vi "GetOutputEnableState.vi"(8 "Error In":errorcluster, 11 "Keithley 6482 In":refnum<visa-resource-name>) -> (0 "Error Out":errorcluster, 2 "Enabled?":bool, 3 "Keithley 6482 Out":refnum<visa-resource-name>)   [LabVIEW 2009, in "Keithley-6482-Visa.lvlib"]
uses:
  <instrlib>/Keithley-6482-Visa9.0/Keithley-6482-Visa.lvlib
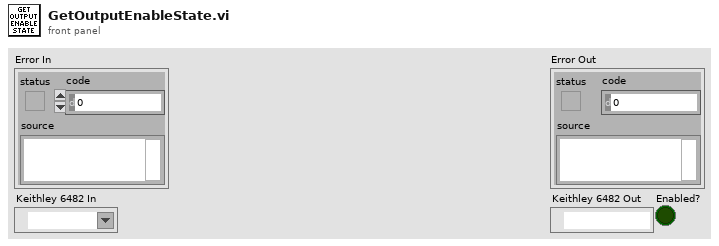
[diagram p1: front panel]
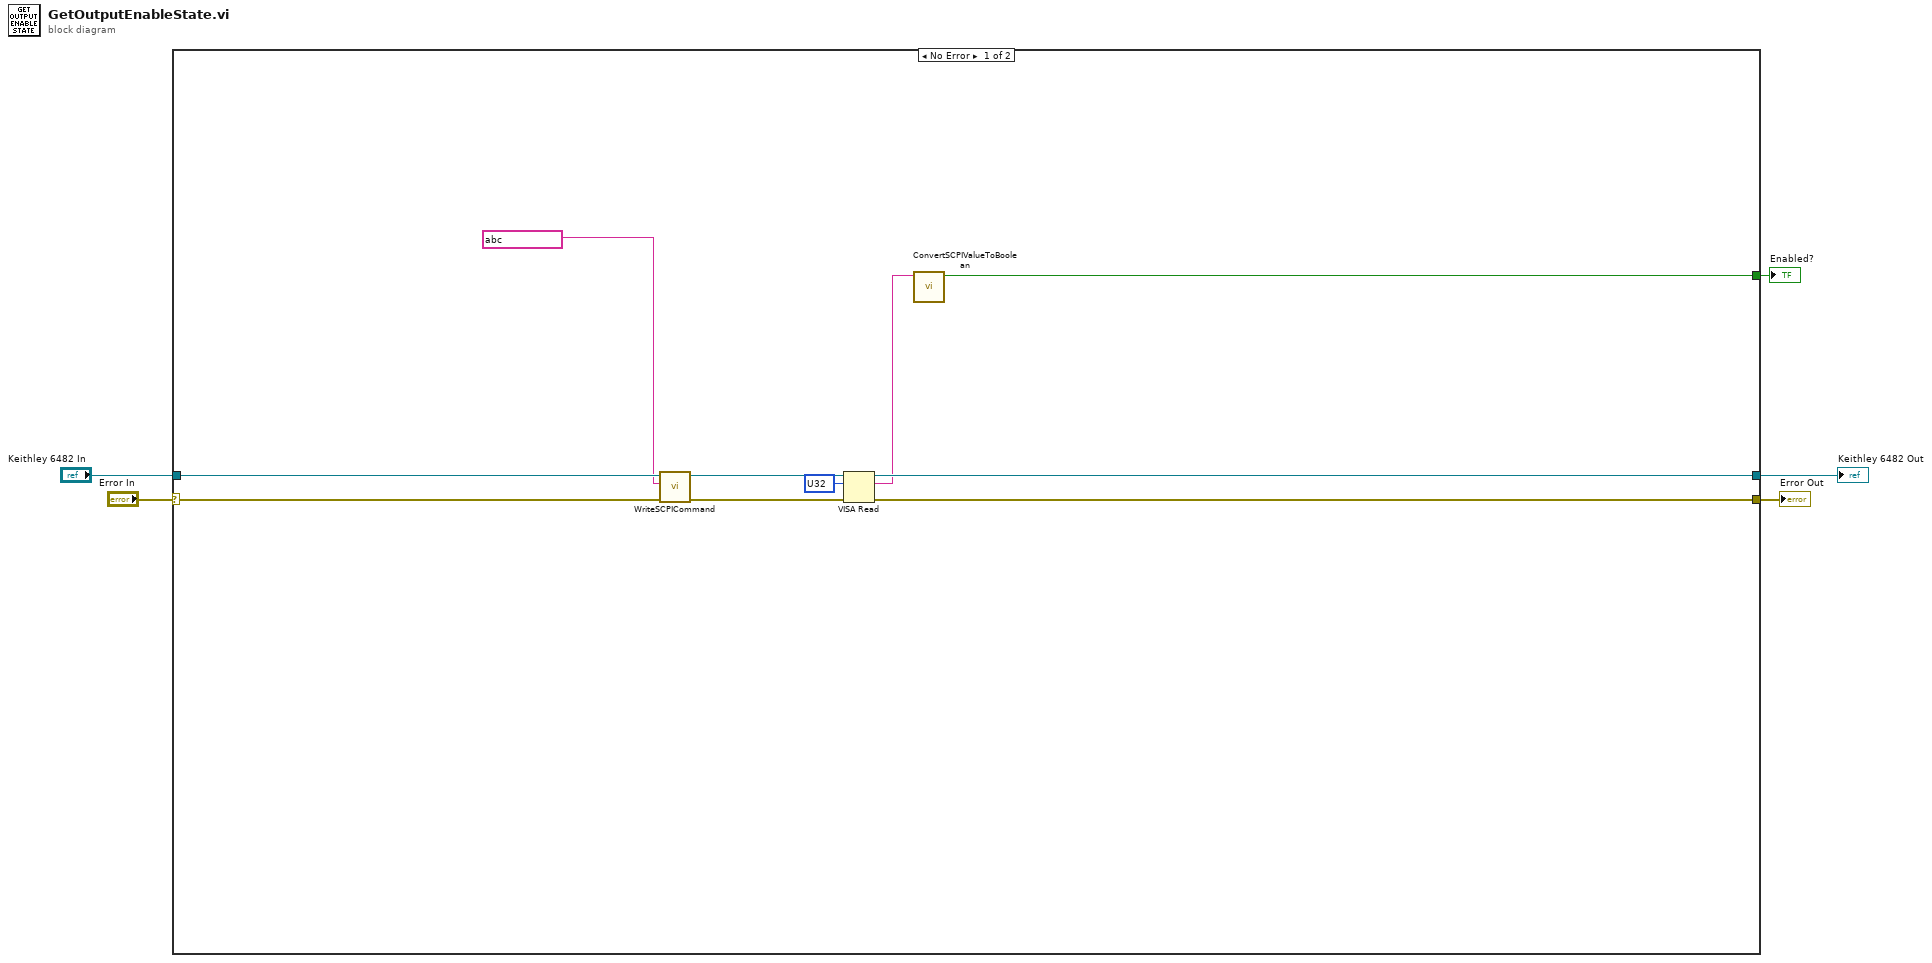
[diagram p0: block diagram]
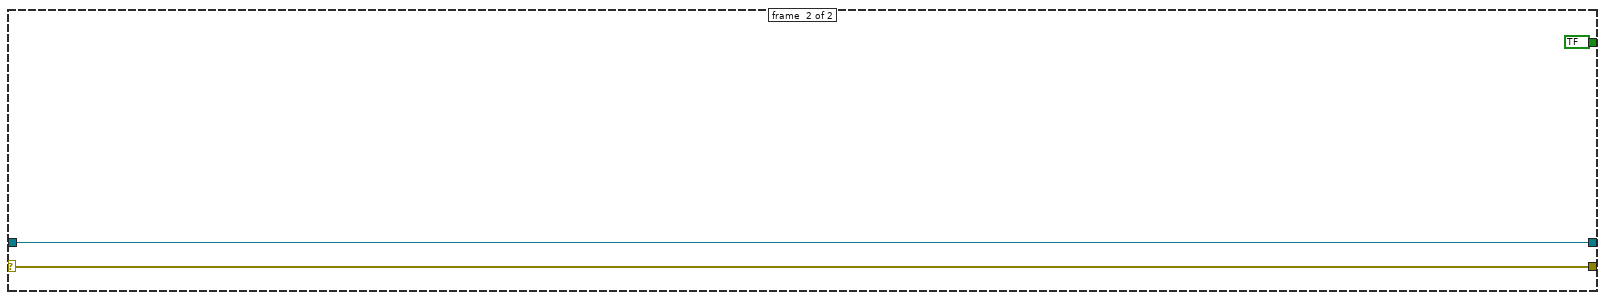
[diagram p2: hidden frame]
diagram:
  n1 = case shown="No Error" "Error In" {
    selector: "Error In" -> [w7 w17]
    tunnel: [w15 w17] -> w4
    tunnel: [w14 w18] -> w3
    tunnel: "Keithley 6482 In" -> [w8 w18]
    tunnel: [w11 bool ? ("Boolean")] -> w1
    frame #0 {
      n2 = call <instrlib>:"WriteSCPICommand.vi"("Error In"=w7, "SCPI Command"=string ?, "Keithley 6482 In"=w8) -> ("Error Out"=w9:errorcluster, "Keithley 6482 Out"=w10:refnum<visa-resource-name>)  [unwired: 7 in]
      n3 = VISA Read(VISA resource name=w10, byte count=u32 ?, error in (no error)=w9) -> (VISA resource name out=w14:refnum<visa-resource-name>, read buffer=w12:string, error out=w15:errorcluster)  [unwired: 1 out]
      n4 = call <instrlib>:"ConvertSCPIValueToBoolean.vi"("SCPI Value"=w12) -> ("Boolean"=w11:bool)  [unwired: 10 in]
    }
    frame #1 {
    }
  }
  "Error Out" <- w4
  "Keithley 6482 Out" <- w3
  "Enabled?" <- w1
